vi "stageGoAbs.vi"(11 "abs pos":dbl) -> ()   [LabVIEW 2016]
uses:
  <vilib>/Instr/_visa.llb/VISA Configure Serial Port (Instr).vi
panel:
  out "Moving":bool
  out "Stage Position":string
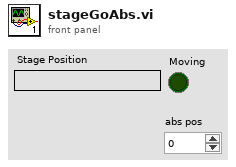
[diagram p1: front panel]
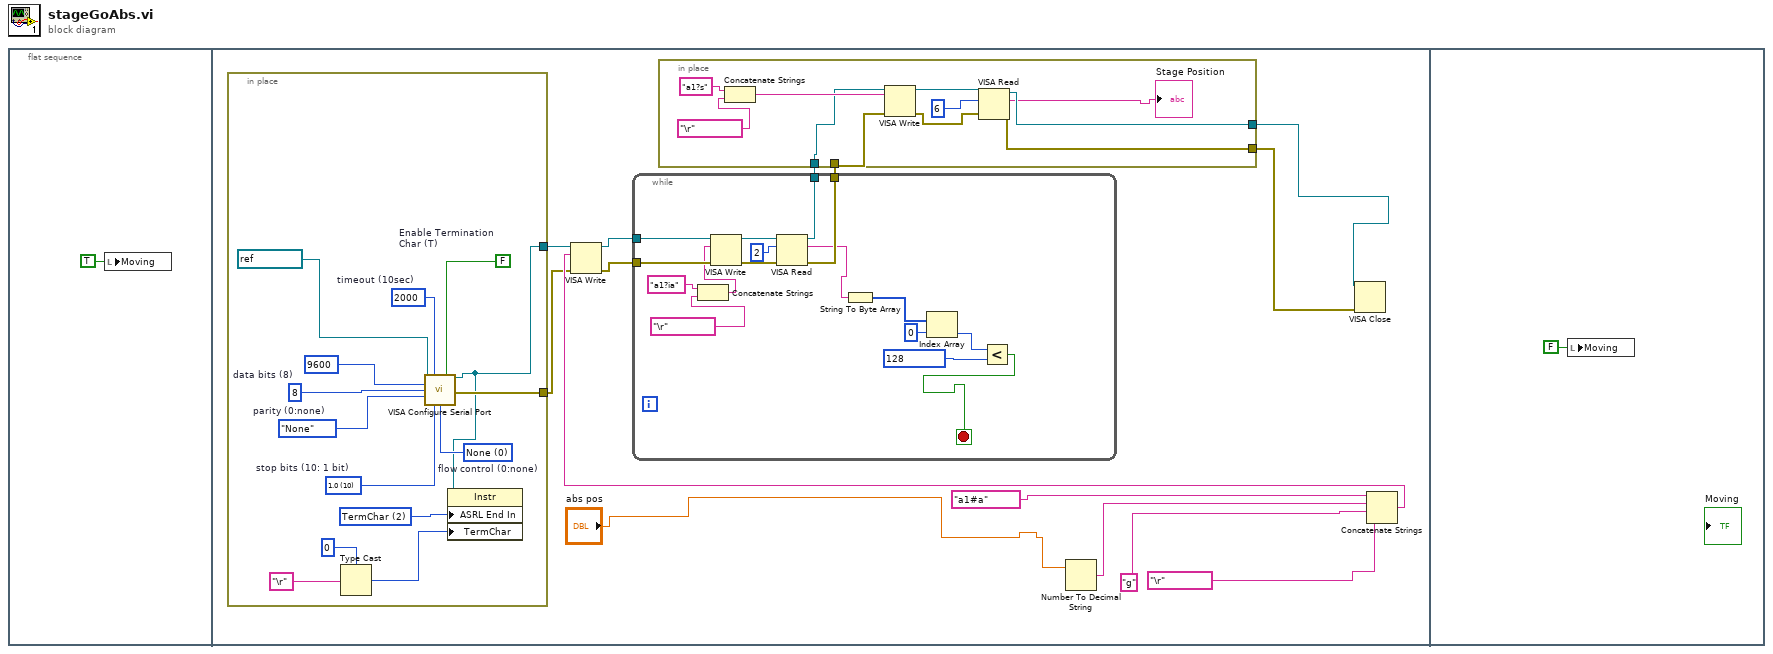
[diagram p0: block diagram]
diagram:
  n1 = flat-sequence {
    frame #0 {
      n2 = local write "Moving"(TRUE ("Moving")) -> ()
    }
    frame #1 {
      n3 = in-place {
        in-place-border: [w27] -> w10
        in-place-border: [w32] -> w9
        w28 = u16 2 items=["None", "Last Bit", "TermChar"] ("Serial Settings:End Mode for Reads")
        w34 = u16 0 items=["None", "XON/XOFF", "RTS/CTS", "XON/XOFF & RTS/CTS", "DTR/DSR", "XON/XOFF & DTR/DSR"]  # flow control (0:none)
        w35 = u16 10 items=["1.0"=10, "1.5"=15, "2.0"=20]  # stop bits (10: 1 bit)
        w36 = FALSE  # Enable Termination Char (T)
        w37 = u32 2000  # timeout (10sec)
        w38 = enum16{"None", "Odd", "Even", "Mark", "Space"}."None"  # parity (0:none)
        w39 = u16 8  # data bits (8)
        n4 = Type Cast(type=u8 0, x="\r") -> (*(type *) &x=w30:u8)
        n5 = call-poly "VISA Configure Serial Port"("VISA resource name"=refnum<visa-resource-name> "COM4", "timeout (10sec)"=w37, "Enable Termination\nChar (T)"=w36, "baud rate (9600)"=u32 9600, "data bits (8)"=w39, "parity (0:none)"=w38, "stop bits (10: 1 bit)"=w35, "flow control (0:none)"=w34) -> ("VISA resource name out"=w27:refnum<visa-resource-name>, "error out"=w32:errorcluster)  [unwired: 6 in]
        n6 = property class="Instr"(reference=w27, "ASRL End In"=w28, "TermChar"=w30) -> ()  [unwired: 1 in, 2 out]
      }
      n7 = Number To Decimal String(number="abs pos") -> (decimal integer string=w14:string)  [unwired: 1 in]
      n8 = Concatenate Strings("a1#a" ("string"), w14, "g" ("string"), "\r" ("write buffer")) -> (w15:string)
      n9 = VISA Write(VISA resource name=w10, write buffer=w15, error in (no error)=w9) -> (VISA resource name out=w8:refnum<visa-resource-name>, error out=w7:errorcluster)  [unwired: 1 out]
      n10 = while {
        tunnel: w8 -> [w56]
        tunnel: w7 -> [w55]
        tunnel: [w48] -> w6
        tunnel: [w47] -> w5
        stop <- w41 stop-if-true
        n11 = Concatenate Strings("a1?ia" ("write buffer"), "\r" ("write buffer")) -> (w52:string)
        n12 = VISA Write(VISA resource name=w56, write buffer=w52, error in (no error)=w55) -> (VISA resource name out=w51:refnum<visa-resource-name>, error out=w50:errorcluster)  [unwired: 1 out]
        n13 = VISA Read(VISA resource name=w51, byte count=u32 2, error in (no error)=w50) -> (VISA resource name out=w48:refnum<visa-resource-name>, read buffer=w46:string, error out=w47:errorcluster)  [unwired: 1 out]
        n14 = String To Byte Array(string=w46) -> (unsigned byte array=w45:u8[])
        n15 = Index Array(array=w45, index=0) -> (element=w43:u8)
        n16 = Less?(x=w43, y=u8 128) -> (x < y?=w41:bool)
      }
      n17 = in-place {
        in-place-border: w6 -> [w21]
        in-place-border: w5 -> [w20]
        in-place-border: [w19] -> w4
        in-place-border: [w18] -> w3
        n18 = Concatenate Strings("a1?s" ("write buffer"), "\r" ("write buffer")) -> (w24:string)
        n19 = VISA Write(VISA resource name=w21, write buffer=w24, error in (no error)=w20) -> (VISA resource name out=w25:refnum<visa-resource-name>, error out=w17:errorcluster)  [unwired: 1 out]
        n20 = VISA Read(VISA resource name=w25, byte count=u32 6, error in (no error)=w17) -> (VISA resource name out=w18:refnum<visa-resource-name>, read buffer=→"Stage Position":string, error out=w19:errorcluster)  [unwired: 1 out]
      }
      n21 = VISA Close(VISA resource name=w3, error in (no error)=w4) -> ()  [unwired: 1 out]
    }
    frame #2 {
      n22 = local write "Moving"(FALSE ("Moving")) -> ()
    }
  }
